vi "UHR-Fleezers Control (host) - 12.5.vi"() -> ()   [LabVIEW 2012] (continued)
            n989 = call "Set Stage Position.vi"("Position"=w1420, "error in"=w1421, "VISA resource name in"=w1422) -> ()  [unwired: 3 out]
          }
          frame #3 {
            # "stop saving"
            n990 = local write "Stop Saving"(TRUE ("Stop Saving")) -> ()
            n991 = local write "Stage Moving"(FALSE ("Stage Moving")) -> ()
          }
        }
      }
      event "Move to Position 1", "Move to Position 2", "Move to Position 3", "Move to Position 4", "Move to Position 5", "Lower Ch. Cap.": Value Change {
        n992 = event-data() -> ()  [unwired: 1 in, 5 out]
        n993 = Or(x="Move to Position 5", y="Lower Ch. Cap.") -> (x .or. y?=w1428:bool)
        n994 = Build Array("Move to Position 1", "Move to Position 2", "Move to Position 3", "Move to Position 4", w1428) -> (w1431:bool[])
        n995 = Boolean Array To Number(Boolean array=w1431) -> (number=w1430:u32)
        n996 = Logarithm Base 2(1:w1430) -> (0:w1429:dbl)
        n997 = flat-sequence {
          tunnel: w1429 -> [w1440]
          tunnel: w1426 -> [w1438]
          tunnel: w1425 -> [w1437]
          frame #0 {
            n998 = local read "Saved Stage Positions"() -> (w1448:dbl[][])
            n999 = Array Subset(array=w1448, index (row)=w1440, length (row)=1 ("length"), index (col)=1 ("index"), length (col)=3 ("length")) -> (w1445:dbl[][])
            n1000 = Reshape Array(w1445, 3 ("dimension size")) -> (w1443:dbl[])
            n1001 = Array To Cluster(array=w1443) -> (cluster=w1442:cluster{"[0]":dbl, "[1]":dbl, "[2]":dbl})
            n1002 = call "Set Stage Position.vi"("Position"=w1442, "error in"=w1437, "VISA resource name in"=w1438) -> ("error out"=w1441:errorcluster)  [unwired: 2 out]
            n1003 = local write "Stage Moving"(TRUE ("Stage Moving")) -> ()
            n1004 = local write "Stage Control Serial Error"(w1441) -> ()
          }
          frame #1 {
            n1005 = local write "Stage Moving"(FALSE ("Stage Moving")) -> ()
            n1006 = call <vilib>:"Beep.vi"() -> ()  [unwired: 3 in, 9 out]
          }
        }
      }
      event "Got ADig bead": Value Change {
        n1007 = event-data() -> ()  [unwired: 1 in, 5 out]
        n1008 = flat-sequence {
          frame #0 {
            n1009 = local read "Cap 1 Samp Flow ON"() -> (w1452:bool)
            n1010 = case shown="True" w1452 {
              frame False {
              }
              frame True {
                n1011 = property on="Sample Channel\nFlow" class="Bool (strict)"("Val(Sgnl)"=TRUE ("Value (Signaling)")) -> ()  [unwired: 2 in, 2 out]
              }
            }
          }
          frame #1 {
            n1012 = property on="Inject Pump 3" class="Bool (strict)"("Val(Sgnl)"=FALSE ("Value (Signaling)")) -> ()  [unwired: 2 in, 2 out]
          }
          frame #2 {
            n1013 = property on="Move Cap. 1 (DNA Bottom)" class="Bool (strict)"("Val(Sgnl)"=TRUE ("Value (Signaling)")) -> ()  [unwired: 2 in, 2 out]
          }
        }
      }
      event "Force FB Data\nScript": Value Change {
        n1014 = event-data() -> ()  [unwired: 1 in, 5 out]
        n1015 = flat-sequence {
          tunnel: w1461 -> [w1465]
          tunnel: w1462 -> [w1466]
          tunnel: [w1466] -> w1457
          tunnel: [w1465] -> w1456
          tunnel: w1457 -> [w1469]
          tunnel: w1456 -> [w1468]
          tunnel: ["Trap Trig Fl."] -> w1458
          tunnel: [w1494] -> w1459
          tunnel: w1458 -> [w1494]
          tunnel: [w1498] -> w1460
          tunnel: w1459 -> [w1498]
          tunnel: w1460 -> [w1500]
          frame #0 {
            n1016 = property on="Trap Delta (MHz)" class="DigNum (strict)"("Val(Sgnl)"="Trap Delta Before Moving") -> ()  [unwired: 2 in, 2 out]
          }
          frame #1 {
            n1017 = local read "Saved Stage Positions"() -> (w1471:dbl[][])
            n1018 = local write "FB Trap Pos Offset"(0.0 ("FB Trap Pos Offset")) -> ()
            n1019 = property on="Trap Pos. FB Offset Factor" class="DigNum (strict)"("Val(Sgnl)"=i64 0 ("Value (Signaling)")) -> ()  [unwired: 2 in, 2 out]
            n1020 = local write "Stage Moving"(TRUE ("Stage Moving")) -> ()
            n1021 = call "move to saved stage position.vi"("error in"=w1468, "Stage VISA resource name in"=w1469, "Position"="Stage Position To Establish FB", "Saved Stage Positions"=w1471) -> ("error out"=w1467:errorcluster)  [unwired: 1 out]
            n1022 = local write "Stage Control Serial Error"(w1467) -> ()
          }
          frame #2 {
            n1023 = call <vilib>:"Beep.vi"() -> ()  [unwired: 3 in, 9 out]
            n1024 = Multiply(x="Wait (s)", y=u32 1000 ("milliseconds to wait")) -> (x*y=w1478:u32)
            n1025 = property on="Trap Delta (MHz)" class="DigNum (strict)"("Val(Sgnl)"="Starting \nTrap Delta (MHz)") -> ()  [unwired: 2 in, 2 out]
            n1026 = local write "Stage Moving"(FALSE ("Stage Moving")) -> ()
            n1027 = Wait (ms)(milliseconds to wait=w1478) -> ()  [unwired: 1 out]
            n1028 = property on="Tab Control 2" class="TabCtl (strict)"("Val(Sgnl)"=T6."Feedback on Trap Position" ("Value (Signaling)")) -> ()  [unwired: 2 in, 2 out]
            n1029 = property on="Tab Control" class="TabCtl (strict)"("Val(Sgnl)"=T4."Trap Control (RF)" ("Value (Signaling)")) -> ()  [unwired: 2 in, 2 out]
          }
          frame #3 {
            n1030 = property on="Set Reading to\nSetpoint" class="Bool (strict)"("Val(Sgnl)"=TRUE ("Value (Signaling)")) -> ()  [unwired: 2 in, 2 out]
            n1031 = Wait (ms)(milliseconds to wait=u32 500) -> ()  [unwired: 1 out]
          }
          frame #4 {
            n1032 = property on="Trap Pos. FB ON" class="Bool (strict)"("Val(Sgnl)"=TRUE ("Value (Signaling)")) -> ()  [unwired: 2 in, 2 out]
            n1033 = Wait (ms)(milliseconds to wait=u32 250) -> ()  [unwired: 1 out]
          }
          frame #5 {
            n1034 = case shown="False" "Trap Trig Fl." {
              frame False {
                n1035 = case shown="True" "Green ON after FB ON?" {
                  selector: "Green ON after FB ON?" -> [_ w1493]
                  frame False {
                  }
                  frame True {
                    n1036 = property on="Green Laser ON" class="Bool (strict)"("Val(Sgnl)"=w1493) -> ()  [unwired: 2 in, 2 out]
                  }
                }
              }
              frame True {
              }
            }
            n1037 = case shown="True" "Remove Action Offset" {
              tunnel: TRUE ("Value (Signaling)") -> [w1490 w1491]
              frame False {
                n1038 = property on="Remove Unwinding Offset" class="Bool (strict)"("Val(Sgnl)"=w1490) -> ()  [unwired: 2 in, 2 out]
              }
              frame True {
                n1039 = property on="Remove Action Offset" class="Bool (strict)"("Val(Sgnl)"=w1491) -> ()  [unwired: 2 in, 2 out]
              }
            }
            n1040 = Wait (ms)(milliseconds to wait=u32 250) -> ()  [unwired: 1 out]
          }
          frame #6 {
            n1041 = property on="Start Saving" class="Bool (strict)"("Val(Sgnl)"=TRUE ("Value (Signaling)")) -> ()  [unwired: 2 in, 2 out]
            n1042 = Wait (ms)(milliseconds to wait=u32 5000) -> ()  [unwired: 1 out]
          }
          frame #7 {
            w1497 = TRUE ("Value (Signaling)")
            n1043 = property on="Rem fb disp offset" class="Bool (strict)"("Val(Sgnl)"=w1497) -> ()  [unwired: 2 in, 2 out]
            n1044 = property on="Remove Offset" class="Bool (strict)"("Val(Sgnl)"=w1497) -> ()  [unwired: 2 in, 2 out]
            n1045 = Wait (ms)(milliseconds to wait=u32 100) -> ()  [unwired: 1 out]
          }
          frame #8 {
            n1046 = case shown="True" w1500 {
              frame False {
              }
              frame True {
                n1047 = local write "Trap Trig. Fl."(TRUE ("Value (Signaling)")) -> ()
              }
            }
          }
          frame #9 {
            n1048 = case shown="True" "Start dipping after?" {
              frame False {
              }
              frame True {
                n1049 = flat-sequence {
                  frame #0 {
                    n1050 = Multiply(x="Delay before dipping (s)", y=1000.0) -> (x*y=w1504:dbl)
                    n1051 = Wait (ms)(milliseconds to wait=w1504) -> ()  [unwired: 1 out]
                  }
                  frame #1 {
                    n1052 = property on="Dip for Protein" class="Bool (strict)"("Val(Sgnl)"=TRUE ("Value (Signaling)")) -> ()  [unwired: 2 in, 2 out]
                    n1053 = local write "Scripts"(T1."Dipping" ("Scripts")) -> ()
                  }
                }
              }
            }
          }
        }
      }
      event "Fixed Traps Data\nScript": Value Change {
        n1054 = event-data() -> ()  [unwired: 1 in, 5 out]
        n1055 = flat-sequence {
          frame #0 {
            n1056 = case shown="True" "Green ON" {
              frame False {
              }
              frame True {
                n1057 = property on="Green Laser ON" class="Bool (strict)"("Val(Sgnl)"=TRUE) -> ()  [unwired: 2 in, 2 out]
              }
            }
            n1058 = local write "Offset (nm)"(0.0 ("Offset (nm)")) -> ()
            n1059 = property on="Sample Channel\nFlow" class="Bool (strict)"("Val(Sgnl)"=FALSE ("Value (Signaling)")) -> ()  [unwired: 2 in, 2 out]
            n1060 = property on="Trap Delta (MHz)" class="DigNum (strict)"("Val(Sgnl)"="Fixed Traps Trap Delta (MHz)") -> ()  [unwired: 2 in, 2 out]
          }
          frame #1 {
            n1061 = Wait (ms)(milliseconds to wait=u32 1000) -> ()  [unwired: 1 out]
          }
          frame #2 {
            n1062 = local write "Start Saving"(TRUE ("Start Saving")) -> ()
          }
          frame #3 {
            n1063 = local read "Bead Sep. Int. Time (s)"() -> (w1515:dbl)
            n1064 = Multiply(x=w1515, y=1000.0) -> (x*y=w1517:dbl)
            n1065 = Wait (ms)(milliseconds to wait=w1517) -> ()  [unwired: 1 out]
          }
          frame #4 {
            n1066 = property on="Remove Offset" class="Bool (strict)"("Val(Sgnl)"=TRUE ("Value (Signaling)")) -> ()  [unwired: 2 in, 2 out]
          }
          frame #5 {
            n1067 = property on="Dip for Protein" class="Bool (strict)"("Val(Sgnl)"="Start dipping after?") -> ()  [unwired: 2 in, 2 out]
          }
        }
      }
      event "Got DNA bead": Value Change {
        n1068 = event-data() -> ()  [unwired: 1 in, 5 out]
        n1069 = flat-sequence {
          frame #0 {
            n1070 = local read "Daq spot flow on"() -> (w1522:bool)
            n1071 = case shown="True" w1522 {
              frame False {
              }
              frame True {
                n1072 = property on="Sample Channel\nFlow" class="Bool (strict)"("Val(Sgnl)"=TRUE ("Value (Signaling)")) -> ()  [unwired: 2 in, 2 out]
              }
            }
            n1073 = property on="Got DNA bead" class="Bool"("Key Focus"=FALSE) -> ()  [unwired: 2 in, 2 out]
          }
          frame #1 {
            n1074 = property on="Inject Pump 1" class="Bool (strict)"("Val(Sgnl)"=FALSE ("Value (Signaling)")) -> ()  [unwired: 2 in, 2 out]
          }
          frame #2 {
            n1075 = property on="Cal/Data Acq. Spot" class="Bool (strict)"("Val(Sgnl)"=TRUE ("Value (Signaling)")) -> ()  [unwired: 2 in, 2 out]
          }
        }
      }
      event "Take Stepping Data": Value Change {
        n1076 = event-data() -> ()  [unwired: 1 in, 5 out]
        n1077 = local read "Save ave N"() -> (w1534:dbl)
        n1078 = flat-sequence {
          tunnel: w1534 -> [w1536]
          tunnel: [w1536] -> w1529
          tunnel: [w1538] -> w1530
          tunnel: w1529 -> [w1538]
          tunnel: [w1540] -> w1531
          tunnel: w1530 -> [w1540]
          tunnel: [w1543] -> w1532
          tunnel: w1531 -> [w1543]
          tunnel: [w1545] -> w1533
          tunnel: w1532 -> [w1545]
          tunnel: [w1547] -> w1527
          tunnel: w1533 -> [w1547]
          tunnel: w1527 -> [w1550]
          tunnel: [w1550] -> w1526
          tunnel: w1526 -> [w1551]
          tunnel: [w1551] -> w1528
          tunnel: w1528 -> [w1557]
          frame #0 {
            n1079 = property on="Save ave N" class="DigNum (strict)"("Val(Sgnl)"="Save ave factor") -> ()  [unwired: 2 in, 2 out]
          }
          frame #1 {
            n1080 = Wait (ms)(milliseconds to wait=u32 100) -> ()  [unwired: 1 out]
          }
          frame #2 {
            n1081 = local read "Offset 2 Start (MHz)"() -> (w1542:dbl)
            n1082 = property on="Saved AOD Raster Scan Parameter Sets" class="Arr (strict)"("Index Values"=u32[] [2]) -> ()  [unwired: 2 in, 2 out]
            n1083 = property on="Trap Delta (MHz)" class="DigNum (strict)"("Val(Sgnl)"=w1542) -> ()  [unwired: 2 in, 2 out]
          }
          frame #3 {
            n1084 = property on="Load parameters" class="Bool (strict)"("Val(Sgnl)"=TRUE ("Value (Signaling)")) -> ()  [unwired: 2 in, 2 out]
          }
          frame #4 {
            n1085 = Wait (ms)(milliseconds to wait=u32 100) -> ()  [unwired: 1 out]
          }
          frame #5 {
            n1086 = property on="Trap Raster Scan" class="Bool (strict)"("Val(Sgnl)"=TRUE ("Value (Signaling)")) -> ()  [unwired: 2 in, 2 out]
          }
          frame #6 {
            n1087 = Wait (ms)(milliseconds to wait=u32 1000) -> ()  [unwired: 1 out]
          }
          frame #7 {
            n1088 = while {
              stop <- w1554 stop-if-true
              n1089 = local read "Raster Scanning..."() -> (w1556:bool)
              n1090 = local read "Saving..."() -> (w1555:bool)
              n1091 = Not(x=w1555) -> (.not. x?=w1552:bool)
              n1092 = Not(x=w1556) -> (.not. x?=w1553:bool)
              n1093 = And(x=w1553, y=w1552) -> (x .and. y?=w1554:bool)
            }
          }
          frame #8 {
            n1094 = property on="Save ave N" class="DigNum (strict)"("Val(Sgnl)"=w1557) -> ()  [unwired: 2 in, 2 out]
          }
        }
      }
      event "Step Size (nm)": Value Change {
        n1095 = event-data() -> ()  [unwired: 1 in, 5 out]
        n1096 = flat-sequence {
          frame #0 {
            n1097 = property on="Saved AOD Raster Scan Parameter Sets" class="Arr (strict)"("Index Values"=u32[] [1]) -> ()  [unwired: 2 in, 2 out]
          }
          frame #1 {
            n1098 = Multiply(x="N Steps", y="Step Size (nm)") -> (x*y=w1559:dbl)
            n1099 = property on="Scan Speed AOD (nm/s) 2" class="DigNum (strict)"("Value"="Step Size (nm)") -> ()  [unwired: 2 in, 2 out]
            n1100 = property on="Step Size AOD (nm) 2" class="DigNum (strict)"("Value"="Step Size (nm)") -> ()  [unwired: 2 in, 2 out]
            n1101 = property on="Scan Range AOD (nm) 2" class="DigNum (strict)"("Value"=w1559) -> ()  [unwired: 2 in, 2 out]
          }
        }
      }
      event "Take Detection Laser\nImage": Value Change {
        n1102 = event-data() -> ()  [unwired: 1 in, 5 out]
        n1103 = flat-sequence {
          tunnel: [w1587] -> w1577
          tunnel: [w1586] -> w1570
          tunnel: [w1585] -> w1562
          tunnel: [w1590] -> w1578
          tunnel: w1577 -> [w1590]
          tunnel: [w1589] -> w1571
          tunnel: w1570 -> [w1589]
          tunnel: [w1588] -> w1563
          tunnel: w1562 -> [w1588]
          tunnel: [w1594] -> w1579
          tunnel: w1578 -> [w1594]
          tunnel: [w1593] -> w1572
          tunnel: w1571 -> [w1593]
          tunnel: [w1592] -> w1564
          tunnel: w1563 -> [w1592]
          tunnel: [w1600] -> w1580
          tunnel: w1579 -> [w1600]
          tunnel: [w1599] -> w1573
          tunnel: w1572 -> [w1599]
          tunnel: [w1598] -> w1565
          tunnel: w1564 -> [w1598]
          tunnel: [w1604] -> w1581
          tunnel: w1580 -> [w1604]
          tunnel: [w1603] -> w1574
          tunnel: w1573 -> [w1603]
          tunnel: [w1602] -> w1566
          tunnel: w1565 -> [w1602]
          tunnel: [w1608] -> w1582
          tunnel: w1581 -> [w1608]
          tunnel: [w1607] -> w1575
          tunnel: w1574 -> [w1607]
          tunnel: [w1606] -> w1567
          tunnel: w1566 -> [w1606]
          tunnel: [w1612] -> w1583
          tunnel: w1582 -> [w1612]
          tunnel: [w1611] -> w1576
          tunnel: w1575 -> [w1611]
          tunnel: [w1610] -> w1568
          tunnel: w1567 -> [w1610]
          tunnel: w1583 -> [w1618]
          tunnel: w1576 -> [w1617]
          tunnel: [w1615] -> w1569
          tunnel: w1568 -> [w1615]
          tunnel: w1569 -> [w1619]
          frame #0 {
            n1104 = local read "Laser interlacing mode"() -> (w1586:enum32{"Laser ON", "Laser OFF", "Interlace"})
            n1105 = local read "Green FB On/Off"() -> (w1585:bool)
            n1106 = local read "Green Laser ON"() -> (w1587:bool)
          }
          frame #1 {
            n1107 = property on="Green FB On/Off" class="Bool (strict)"("Val(Sgnl)"=FALSE ("Value (Signaling)")) -> ()  [unwired: 2 in, 2 out]
          }
          frame #2 {
            n1108 = property on="Green Laser ON" class="Bool (strict)"("Val(Sgnl)"=TRUE ("Value (Signaling)")) -> ()  [unwired: 2 in, 2 out]
            n1109 = property on="Flip Green Filter" class="Bool (strict)"("Val(Sgnl)"=TRUE ("Value (Signaling)")) -> ()  [unwired: 2 in, 2 out]
            n1110 = property on="Laser interlacing mode" class="RadioBtnsControl (strict)"("Val(Sgnl)"=enum32{"Laser ON", "Laser OFF", "Interlace"}."Laser ON" ("Value (Signaling)")) -> ()  [unwired: 2 in, 2 out]
          }
          frame #3 {
            n1111 = Wait (ms)(milliseconds to wait=u32 500) -> ()  [unwired: 1 out]
          }
          frame #4 {
            n1112 = property on="Confocal Image" class="Bool (strict)"("Val(Sgnl)"=TRUE ("Value (Signaling)")) -> ()  [unwired: 2 in, 2 out]
          }
          frame #5 {
            n1113 = Wait (ms)(milliseconds to wait=u32 2000) -> ()  [unwired: 1 out]
          }
          frame #6 {
            n1114 = while {
              stop <- w1613 stop-if-true
              n1115 = local read "Saving..."() -> (w1614:bool)
              n1116 = Not(x=w1614) -> (.not. x?=w1613:bool)
            }
          }
          frame #7 {
            n1117 = property on="Flip Green Filter" class="Bool (strict)"("Val(Sgnl)"=TRUE ("Value (Signaling)")) -> ()  [unwired: 2 in, 2 out]
            n1118 = property on="Green Laser ON" class="Bool (strict)"("Val(Sgnl)"=w1618) -> ()  [unwired: 2 in, 2 out]
            n1119 = property on="Laser interlacing mode" class="RadioBtnsControl (strict)"("Val(Sgnl)"=w1617) -> ()  [unwired: 2 in, 2 out]
          }
          frame #8 {
            n1120 = property on="Green FB On/Off" class="Bool (strict)"("Val(Sgnl)"=w1619) -> ()  [unwired: 2 in, 2 out]
          }
        }
      }
      event "Stop All": Value Change {
        n1121 = event-data() -> ()  [unwired: 1 in, 5 out]
        n1122 = local read "Delay (ms)"() -> (w1622:i32)
        n1123 = call "serial write macro.vi"("String"="l0", "Delay (ms)"=w1622, "VISA resource name"=w1625) -> ("read buffer"=w1620:string, "error out"=w1621:errorcluster, "VISA resource name out"=w1624:refnum<visa-resource-name>)
        n1124 = local write "read blue buffer"(w1620) -> ()
        n1125 = local write "Blue Error Out"(w1621) -> ()
        n1126 = VISA Close(VISA resource name=w1624) -> ()  [unwired: 1 in, 1 out]
        n1127 = local read "Stop All"() -> (w1626:bool)
      }
    }
    n1128 = node-c288() -> ()  [unwired: 1 in, 1 out]
  }
  n1129 = timed-loop "Basic control parameters (all FPGA settings, other basic controls)" {
    tunnel: w13 -> [w1635]
    shift-right: [w1634] -> _
    shift-left: errorcluster {"status"=FALSE, "code"=0, "source"=""} ("error out") -> [w1633]
    tunnel: [w1632] -> _
    timing: w127 -> [_]
    timing-out: [_] -> w126
    tunnel: w100 -> [w1631]
    tunnel: w72 -> [w1630]
    tunnel: w71 -> [w1629]
    tunnel: w70 -> [w1628]
    tunnel: w69 -> [w1627]
    stop <- w1632 stop-if-true
    n1130 = node-c288() -> ()  [unwired: 2 out]
    n1131 = event shown="[0] \"AI Count (ticks)\", \"Sets to FIFO (Traps)\", \"Save ave N\", \"FPGA Ave.\", \"# Samples/channel\", \"N sets to save\": Value Change" {
      selector: _ -> [_ _ _ _ _ _ _ _ _ _ _ _ _ _ _ _ _ _ _ _ _ _ _ _ _ _ _ _ _ _ _ _ _ _ _ _ _ _ _ _ _ _ _ _ _ _ _ _ _ _ _ _ _ _ _ _ _ _ _ _ _ _ _ _ _ _ _ _ _ _ _ _ _ _]
      dyn-events: _ -> [_ _ _ _ _ _ _ _ _ _ _ _ _ _ _ _ _ _ _ _ _ _ _ _ _ _ _ _ _ _ _ _ _ _ _ _ _ _ _ _ _ _ _ _ _ _ _ _ _ _ _ _ _ _ _ _ _ _ _ _ _ _ _ _ _ _ _ _ _ _ _ _ _ _]
      timeout: _ -> [_ _ _ _ _ _ _ _ _ _ _ _ _ _ _ _ _ _ _ _ _ _ _ _ _ _ _ _ _ _ _ _ _ _ _ _ _ _ _ _ _ _ _ _ _ _ _ _ _ _ _ _ _ _ _ _ _ _ _ _ _ _ _ _ _ _ _ _ _ _ _ _ _ _]
      tunnel: w1635 -> [w1676 _ _ _ w1714 _ w1736 _ _ _ _ w1802 _ _ w1845 w1851 w1858 w1863 w1954 _ w1970 w1995 w2016 w2037 w2058 w2087 w2113 w2116 w2120 w2215 w2220 w2258 _ w2293 w2297 w2308 w2312 w2316 _ w2324 _ _ _ _ _ _ _ _ _ _ _ _ _ _ _ _ _ w2702 _ w2719 _ w2726 w2744 _ w2751 w2759 w2774 w2790 w2796 _ w2805 _ w2824 _]
      tunnel: [w1675 _ _ _ w1704 _ w1735 _ _ w1767 _ w1781 _ _ w1844 w1847 w1857 w1860 w1948 _ w1969 w1994 w2014 w2035 w2056 w2081 w2111 _ w2118 w2213 w2218 w2256 _ w2291 w2295 w2299 w2310 w2314 _ w2322 _ _ _ _ _ _ _ _ _ _ _ _ _ _ _ _ _ w2700 _ _ _ _ w2741 _ _ _ _ _ _ _ _ _ _ _] -> w1634
      tunnel: w1633 -> [w1674 _ _ _ w1713 _ w1734 _ _ w1767 _ w1801 _ _ w1843 w1846 w1856 w1859 w1953 _ w1968 w1993 w2015 w2036 w2057 w2086 w2112 w2115 w2119 w2214 w2219 w2257 _ w2292 w2296 w2307 w2311 w2315 _ w2323 _ _ _ _ _ _ _ _ _ _ _ _ _ _ _ _ _ w2701 _ w2718 _ w2725 w2743 _ w2750 w2758 w2773 w2789 w2795 _ w2804 _ w2823 _]
      tunnel: [_ _ _ _ _ _ _ _ _ w1766 _ _ _ _ _ _ _ _ _ _ _ _ _ _ _ _ _ _ _ _ _ _ _ _ _ _ _ _ _ _ _ _ _ _ _ _ _ _ _ _ _ _ _ _ _ _ _ _ _ _ _ _ _ _ _ _ _ _ _ _ _ _ _ _] -> w1632
      tunnel: [_ _ _ _ _ _ _ "Round T1 X" _ _ _ _ _ _ _ _ _ _ _ _ _ _ _ _ _ _ _ _ _ _ _ _ _ _ _ _ _ _ _ _ _ _ _ _ _ _ _ _ _ _ _ _ _ _ _ _ _ _ _ _ _ _ _ _ _ _ _ _ _ _ _ _ _ _] -> _
      tunnel: [_ _ _ "Adjust Scale\nto Mean" _ _ _ _ _ _ _ _ _ _ _ _ _ _ _ _ _ _ _ _ _ _ _ _ "Test ttrig" _ _ _ _ _ _ _ _ _ _ _ _ _ _ _ _ _ _ "Flush Sample" "Flush Pump 3" "Flush Pump 1" "Clear Volume" _ _ _ _ _ _ _ _ _ _ _ _ _ _ _ _ _ _ _ _ _ _ _] -> _
      tunnel: [_ _ _ _ _ _ _ _ "Round T2 X" _ "Delayed Interlace Start" _ _ _ _ _ _ _ _ _ _ _ _ _ _ _ _ _ _ _ _ _ _ _ _ _ _ _ _ _ _ _ _ _ _ _ _ _ _ _ _ _ _ _ _ _ _ _ _ _ _ _ _ _ _ _ _ _ _ _ _ _ _ _] -> _
      tunnel: w1631 -> [_ _ _ _ _ _ _ _ _ _ _ _ _ _ _ _ _ _ _ _ _ _ _ _ _ _ _ _ _ _ _ _ _ _ _ _ _ _ _ _ _ _ _ w2481 w2488 w2495 w2500 w2509 _ _ w2615 _ _ _ _ _ _ _ _ _ _ _ _ _ _ _ _ _ _ _ _ _ _ _]
      tunnel: w1630 -> [_ _ _ _ _ _ _ _ _ _ _ _ _ _ _ _ _ _ _ _ _ _ _ _ _ _ _ _ _ _ _ _ _ _ _ _ _ _ _ _ _ w2398 _ _ _ _ _ _ w2553 _ _ w2621 _ w2630 _ w2644 _ _ _ _ _ _ _ _ _ _ _ _ _ _ _ _ _ _]
      tunnel: w1629 -> [_ _ _ _ _ _ _ _ _ _ _ _ _ _ _ _ _ _ _ _ _ _ _ _ _ _ _ _ _ _ _ _ _ _ _ _ _ _ _ _ _ _ _ _ _ _ _ _ _ _ _ _ _ _ _ _ _ _ _ _ _ _ _ _ _ _ _ _ _ _ _ _ _ _]
      tunnel: w1628 -> [_ _ _ _ _ _ _ _ _ _ _ _ _ _ _ _ _ _ _ _ _ _ _ _ _ _ _ _ _ _ _ _ _ _ _ _ _ _ _ _ w2335 _ _ _ _ _ _ _ _ w2583 _ _ w2626 _ w2637 _ w2669 _ _ _ _ _ _ _ _ _ _ _ _ _ _ _ _ _]
      tunnel: w1627 -> [_ _ _ _ _ _ _ _ _ _ _ _ _ _ _ _ _ _ _ _ _ _ _ _ _ _ _ _ _ _ _ _ _ _ _ _ _ _ _ _ _ _ _ _ _ _ _ _ _ _ _ _ _ _ _ _ _ _ _ _ _ _ _ _ _ _ _ _ _ _ _ _ _ _]
      event "AI Count (ticks)", "Sets to FIFO (Traps)", "Save ave N", "FPGA Ave.", "# Samples/channel", "N sets to save": Value Change {
        # "So that if 'Save ave N' is updated, the AOD scanning code updates too."
        n1132 = event-data() -> ()  [unwired: 6 out]
        n1133 = local read "AI Count (ticks)"() -> (w1658:u16)
        n1134 = Unbundle By Name("Sets to FIFO (Traps)") -> ("Set 1"=w1641:bool, "Set 2"=w1640:bool, "Set 3"=w1639:bool)
        n1135 = Boolean To (0,1)(Boolean="Sets to FIFO (Traps)") -> (0, 1=w1666:cluster{"Set 1":i16, "Set 2":i16, "Set 3":i16})
        n1136 = xnode "Read/Write Control"("FPGA VI Reference In"=w1676, "error in"=w1674, "ai count"=w1658, "Set 1"=w1641, "Set 2"=w1640, "Set 3"=w1639, "N of AI1 Int Acq Sets"="N Acq Sets (Traps + Fl.)") -> ("error out"=w1675:errorcluster)  [unwired: 1 out]
        n1137 = Cluster To Array(cluster=w1666) -> (array=w1665:i16[])
        n1138 = To Unsigned Long Integer(number=w1665) -> (unsigned 32bit integer=w1647:u32[])
        n1139 = local read "Scan steps (AOD)"() -> (w1667:u64)
        n1140 = Multiply(x=w1658, y="N Acq Sets (Traps + Fl.)") -> (x*y=w1656:u16)
        n1141 = Divide(x=40000000.0, y=w1658) -> (x/y=w1650:dbl)
        "AI rate (Hz)" <- w1650
        "Ave. Rate (Hz)" <- w1650
        n1142 = Add Array Elements(numeric array=w1647) -> (sum=w1659:u32)
        "Trap Sets" <- w1659
        n1143 = Reciprocal(x=w1650) -> (1/x=→"Ave. Period (s)":dbl)
        n1144 = property on="Scan steps (AOD)" class="DigNum (strict)"("Val(Sgnl)"=w1667) -> ()  [unwired: 2 in, 2 out]
        n1145 = Divide(x=w1650, y="N Acq Sets (Traps + Fl.)") -> (x/y=w1671:dbl)
        "Data Rate (Hz)" <- w1671
        n1146 = Reciprocal(x=w1671) -> (1/x=→"Data Period (s)":dbl)
        n1147 = local read "Save ave N"() -> (w1670:dbl)
        n1148 = Divide(x=w1671, y=w1670) -> (x/y=w1669:dbl)
        "Save Data Rate (Hz)" <- w1669
        n1149 = Reciprocal(x=w1669) -> (1/x=→"Save Data Period (s)":dbl)
        n1150 = Multiply(x=w1656, y="# Samples/trap") -> (x*y=w1654:u32)
        "Counts/DMA" <- w1654
        n1151 = property on="Trap Disp. Downsample" class="DigNum (strict)"("Maximum"="# Samples/trap") -> ()  [unwired: 2 in, 2 out]
        n1152 = Multiply(x=w1659, y="# Samples/trap") -> (x*y=w1648:u32)
        "# Samples/channel" <- w1648
        n1153 = Multiply(x=w1648, y=u32 8) -> (x*y=→"Trap AI Elements/DMA read":u32)
        n1154 = local read "APD Int. Count"() -> (w1655:u32)
        n1155 = Multiply(x=w1648, y=u32 3) -> (x*y=→"Trap Pos Elements/DMA read":u32)
        n1156 = Divide(x=w1654, y=w1655) -> (x/y=w1645:dbl)
        "APD Samples/FIFO Acq." <- w1645
        n1157 = Divide(x=w1654, y=40000000.0) -> (x/y=w1652:dbl)
        "DMA Update Period (s)" <- w1652
        n1158 = local read "Number of APDs"() -> (w1638:u8)
        n1159 = Multiply(x=w1638, y=w1645) -> (x*y=→"APD Elements/DMA read":dbl)
        n1160 = property on="APD Disp. Downsample" class="DigNum (strict)"("Maximum"=w1645) -> ()  [unwired: 2 in, 2 out]
        n1161 = local read "N sets to save"() -> (w1664:u32)
        n1162 = Multiply(x=w1652, y=w1664) -> (x*y=→"Total Time (s)":dbl)
        "FPGA Averaging" <- FALSE ("FPGA Averaging")
      }
      event "Remove Offset": Value Change {
        n1163 = event-data() -> ()  [unwired: 7 out]
        n1164 = local write "Remove Offset"(FALSE ("Remove Offset")) -> ()
        n1165 = local read "Bead Mean (nm)"() -> (w1678:dbl)
        n1166 = local read "Offset (nm)"() -> (w1679:dbl)
        n1167 = Add(x=w1678, y=w1679) -> (x+y=w1677:dbl)
        n1168 = local write "Offset (nm)"(w1677) -> ()
        n1169 = disable-structure shown="Disabled" {
          frame Disabled {
            n1170 = local read "Bead Mean (nm)"() -> (w1684:dbl)
            n1171 = Add(y=w1684) -> (x=w1683:dbl, x+y=w1682:dbl)
            n1172 = Subtract(x=w1684, y=w1683) -> (x-y=w1681:dbl)
            n1173 = property on="Bead Separation" class="WFChart (strict)"("YScale.Minimum"=w1681) -> ()  [unwired: 2 in, 2 out]
            n1174 = property on="Bead Separation" class="WFChart (strict)"("YScale.Maximum"=w1682) -> ()  [unwired: 2 in, 2 out]
          }
          frame Enabled {
          }
        }
      }
      event "Detector Type": Value Change {
        n1175 = event-data() -> ()  [unwired: 7 out]
        n1176 = local read "AI labels"() -> (w1685:string[])
        n1177 = property on="High Res. Display" class="Ring (strict)"("Strings []"=w1685) -> ()  [unwired: 2 in, 2 out]
        n1178 = Build Array (concatenate)(w1685, "none") -> (w1686:string[])
        n1179 = property on="FFT 1 Choice 1" class="Ring (strict)"("Strings []"=w1686) -> ()  [unwired: 2 in, 2 out]
        n1180 = property on="FFT 1 Choice 2" class="Ring (strict)"("Strings []"=w1686) -> ()  [unwired: 2 in, 2 out]
        n1181 = property on="FFT 2 Choice 1" class="Ring (strict)"("Strings []"=w1686) -> ()  [unwired: 2 in, 2 out]
        n1182 = property on="FFT 2 Choice 2" class="Ring (strict)"("Strings []"=w1686) -> ()  [unwired: 2 in, 2 out]
        n1183 = Bundle("APD 1", "APD 2") -> (w1689:cluster{string, string})  [unwired: 1 out]
        n1184 = Cluster To Array(cluster=w1689) -> (array=w1687:string[])
        n1185 = Build Array (concatenate)(w1687, w1686) -> (w1691:string[])
        n1186 = Array Size(array=w1691) -> (size(s)=w1692:i32)
        n1187 = property on="Signals to Plot" class="LstBox (strict)"("Item Names"=w1691) -> ()  [unwired: 2 in, 2 out]
        n1188 = property on="Signals to Plot" class="LstBox (strict)"("Number of Rows"=w1692) -> ()  [unwired: 2 in, 2 out]
        n1189 = property on="All Signals" class="WFChart (strict)"("LegNumRows"=w1692) -> ()  [unwired: 2 in, 2 out]
      }
      event "Adjust Scale\nto Mean": Value Change {
        n1190 = event-data() -> ()  [unwired: 7 out]
        n1191 = local read "APD 1 Rate (Hz)"() -> (w1701:dbl)
        n1192 = Multiply(x=1000.0, y="Above (kHz)") -> (x*y=w1699:dbl)
        n1193 = Multiply(x=1000.0, y="Below (kHz)") -> (x*y=w1697:dbl)
        n1194 = Add(x=w1699, y=w1701) -> (x+y=w1694:dbl)
        n1195 = Subtract(x=w1701, y=w1697) -> (x-y=w1695:dbl)
        n1196 = property on="APD Chart" class="WFChart (strict)"("YScale.Minimum"=w1695) -> ()  [unwired: 2 in, 2 out]
        n1197 = property on="APD Chart" class="WFChart (strict)"("YScale.Maximum"=w1694) -> ()  [unwired: 2 in, 2 out]
      }
      event "Phase adj. (AI1)", "+ phase (AI1)", "- phase (AI1)": Value Change {
        n1198 = event-data() -> ()  [unwired: 7 out]
        n1199 = Negate(x="Phase adj. (AI1)") -> (-x=w1711:i16)
        n1200 = Select(t=w1711, s="- phase (AI1)", f="Phase adj. (AI1)") -> (s? t:f=w1710:i16)
        n1201 = xnode "Read/Write Control"("FPGA VI Reference In"=w1714, "error in"=w1713, "Phase count adjustment"=w1710) -> ("FPGA VI Reference Out"=w1709:T20, "error out"=w1708:errorcluster)
        n1202 = Or(x="- phase (AI1)", y="+ phase (AI1)") -> (x .or. y?=w1705:bool)
        n1203 = xnode "Read/Write Control"("FPGA VI Reference In"=w1709, "error in"=w1708, "+ phase"=w1705) -> ("error out"=w1704:errorcluster)  [unwired: 1 out]
      }
      event "Signals to Plot": Double Click {
        w1717 = u32 9868950 ("Color Box")
        n1204 = event-data() -> ("Row"=w1719:i32)  [unwired: 9 out]
        n1205 = property on="All Signals" class="WFChart (strict)"("Active Plot"=w1719) -> (error out=w1730:errorcluster)  [unwired: 2 in, 1 out]
        n1206 = property on="All Signals" class="WFChart (strict)" props=["Plot", "Visible?", "Plot", "Plot Color"](error in=w1730) -> (error out=w1729:errorcluster, "Plot.Visible?"=w1728:bool)  [unwired: 1 in, 2 out]
        n1207 = Select(t=FALSE ("Plot.Visible"), s=w1728, f=TRUE ("Plot.Visible")) -> (s? t:f=w1723:bool)
        n1208 = property on="All Signals" class="WFChart (strict)"(error in=w1729, "Plot.Visible?"=w1723) -> (error out=w1725:errorcluster)  [unwired: 1 in, 1 out]
        n1209 = property on="All Signals" class="WFChart (strict)"(error in=w1725) -> (error out=w1720:errorcluster, "Plot.Plot Color"=w1724:u32)  [unwired: 1 in, 1 out]
        n1210 = property on="Signals to Plot" class="LstBox (strict)"(error in=w1720, "Active Row"=w1719) -> (error out=w1718:errorcluster)  [unwired: 1 in, 1 out]
        n1211 = Select(t=w1724, s=w1723, f=u32 0) -> (s? t:f=w1721:u32)
        n1212 = property on="Signals to Plot" class="LstBox (strict)"(error in=w1718, "CellFontColor"=w1721, "SelColor"=w1717, "CellBG"=w1717, "CellFontSize"=u32 20 ("Active Row:Cell Font:Size"), "CellFontBold"=TRUE ("Active Row:Cell Font:Bold")) -> ()  [unwired: 1 in, 2 out]
      }
      event "BD 1 Frequency 1 (MHz)", "BD 1 Frequency 2 (MHz)", "BD 1 Frequency 3 (MHz)", "BD 2 Frequency 1 (MHz)", "BD 2 Frequency 2 (MHz)", "BD 2 Frequency 3 (MHz)", "Trap Delta (MHz)": Value Change {
        n1213 = event-data() -> ("CtlRef"=w1733:refnum<vi>)  [unwired: 6 out]
        n1214 = control-ref of="Trap Delta (MHz)"() -> (w1732:refnum<vi>)
        n1215 = Equal?(x=w1732, y=w1733) -> (x = y?=w1731:bool)
        n1216 = case shown="False" "Oscillate Set 1" {
          tunnel: w1736 -> [w1756 _]
          tunnel: [w1755 w1759] -> w1735
          tunnel: w1734 -> [w1754 w1759]
          tunnel: w1731 -> [w1739 _]
          frame False {
            n1217 = local read "BD 1 Frequency 2 (MHz)"() -> (w1743:dbl)
            n1218 = local read "BD 1 Frequency 1 (MHz)"() -> (w1741:dbl)
            n1219 = Subtract(x=w1743, y="Trap Delta (MHz)") -> (x-y=w1740:dbl)
            n1220 = Select(t=w1740, s=w1739, f=w1741) -> (s? t:f=w1738:dbl)
            n1221 = local read "Y RF Frequency Limits (MHz)"() -> (w1744:T16)
            n1222 = local read "X RF Frequency Limits (MHz)"() -> (w1745:T16)
            n1223 = local read "BD 1 Frequency 3 (MHz)"() -> (w1757:dbl)
            n1224 = local write "BD 1 Frequency 1 (MHz)"(w1738) -> ()
            n1225 = local read "BD 2 Frequency 1 (MHz)"() -> (w1748:dbl)
            n1226 = local read "BD 2 Frequency 2 (MHz)"() -> (w1747:dbl)
            n1227 = local read "BD 2 Frequency 3 (MHz)"() -> (w1758:dbl)
            n1228 = call "set RF board frequency - interlace.vi"("Board 2 Frequency Limits"=w1744, "Board 1 Frequency Limits"=w1745, "error in"=w1754, "FPGA VI Reference In"=w1756, "Board 2 Frequency 3 (MHz)"=w1758, "Board 1 Frequency 3 (MHz)"=w1757, "Board 2 Frequency 2 (MHz)"=w1747, "Board 2 Frequency 1 (MHz)"=w1748, "Board 1 Frequency 2 (MHz)"=w1743, "Board 1 Frequency 1  (MHz)"=w1738) -> ("error out"=w1755:errorcluster)  [unwired: 1 out]
            n1229 = Subtract(x=w1748, y=w1747) -> (x-y=w1752:dbl)
            n1230 = Subtract(x=w1738, y=w1743) -> (x-y=w1753:dbl)
            n1231 = Square(x=w1752) -> (x^2=w1750:dbl)
            n1232 = Square(x=w1753) -> (x^2=w1751:dbl)
            n1233 = Add(x=w1751, y=w1750) -> (x+y=w1749:dbl)
            n1234 = Square Root(x=w1749) -> (sqrt(x)=w1746:dbl)
            n1235 = local write "Trap Delta (MHz)"(w1746) -> ()
            n1236 = property on="Initial delta (MHz)" class="DigNum (strict)"("Val(Sgnl)"=w1746) -> ()  [unwired: 2 in, 2 out]
          }
          frame True {
          }
        }
      }
      event "Round T1 X": Value Change {
        n1237 = event-data() -> ()  [unwired: 7 out]
        n1238 = local read "BD 1 Frequency 1 (MHz)"() -> (w1762:dbl)
        n1239 = Round To Nearest(number=w1762) -> (nearest integer value=w1761:dbl)
        n1240 = property on="BD 1 Frequency 1 (MHz)" class="DigNum (strict)"("Val(Sgnl)"=w1761) -> ()  [unwired: 2 in, 2 out]
      }
      event "Round T2 X": Value Change {
        n1241 = event-data() -> ()  [unwired: 7 out]
        n1242 = local read "BD 1 Frequency 2 (MHz)"() -> (w1764:dbl)
        n1243 = Round To Nearest(number=w1764) -> (nearest integer value=w1763:dbl)
        n1244 = property on="BD 1 Frequency 2 (MHz)" class="DigNum (strict)"("Val(Sgnl)"=w1763) -> ()  [unwired: 2 in, 2 out]
      }
      event "Stop All": Value Change {
        n1245 = event-data() -> ()  [unwired: 7 out]
        n1246 = local read "Stop All"() -> (w1766:bool)
      }
      event "Delayed Interlace Start": Value Change {
        n1247 = event-data() -> ()  [unwired: 7 out]
        n1248 = flat-sequence {
          frame #0 {
            n1249 = Multiply(x="Delay to Interlace (s)", y=1000.0) -> (x*y=w1769:dbl)
            n1250 = Wait (ms)(milliseconds to wait=w1769) -> ()  [unwired: 1 out]
          }
          frame #1 {
            n1251 = property on="Laser interlacing mode" class="RadioBtnsControl (strict)"("Val(Sgnl)"=enum32{"Laser ON", "Laser OFF", "Interlace"}."Interlace" ("Value (Signaling)")) -> ()  [unwired: 2 in, 2 out]
          }
        }
      }
      event "BD 1 Amplitude 1 (%)", "BD 1 Amplitude 2 (%)", "BD 1 Amplitude 3 (%)", "BD 2 Amplitude 1 (%)", "BD 2 Amplitude 2 (%)", "BD 2 Amplitude 3 (%)", "Trap 1 ON", "Trap 2 ON", "Trap 3 ON", "Feedback On/Off", "All FB On/Off": Value Change {
        w1793 = i16 1 ("f")
        n1252 = event-data() -> ()  [unwired: 7 out]
        n1253 = local write "Trap 1 (ON/OFF)"("Trap 1 ON") -> ()
        n1254 = local write "Trap 2 (ON/OFF)"("Trap 2 ON") -> ()
        n1255 = Boolean To (0,1)(Boolean="Trap 3 ON") -> (0, 1=w1794:i16)
        n1256 = Boolean To (0,1)(Boolean="Trap 1 ON") -> (0, 1=w1795:i16)
        n1257 = Boolean To (0,1)(Boolean="Trap 2 ON") -> (0, 1=w1796:i16)
        n1258 = Select(t=w1796, s="Trap ON/OFF X or Y Amp?", f=w1793) -> (s? t:f=w1791:i16)
        n1259 = Select(t=w1795, s="Trap ON/OFF X or Y Amp?", f=w1793) -> (s? t:f=w1792:i16)
        n1260 = Select(t=w1794, s="Trap ON/OFF X or Y Amp?", f=w1793) -> (s? t:f=w1790:i16)
        n1261 = Select(t=w1793, s="Trap ON/OFF X or Y Amp?", f=w1796) -> (s? t:f=w1788:i16)
        n1262 = Select(t=w1793, s="Trap ON/OFF X or Y Amp?", f=w1795) -> (s? t:f=w1789:i16)
        n1263 = Select(t=w1793, s="Trap ON/OFF X or Y Amp?", f=w1794) -> (s? t:f=w1787:i16)
        n1264 = And(x="All FB On/Off", y="Feedback On/Off") -> (x .and. y?=w1785:cluster{"Set 1":bool, "Set 2":bool})
        n1265 = local read "BD 1 Amplitude 1 (%)"() -> (w1805:dbl)
        n1266 = local read "BD 1 Amplitude 2 (%)"() -> (w1804:dbl)
        n1267 = local read "BD 1 Amplitude 3 (%)"() -> (w1803:dbl)
        n1268 = Unbundle By Name(w1785) -> ("Set 1"=w1780:bool, "Set 2"=w1777:bool)
        n1269 = local read "Y RF Amplitude Limits (%)"() -> (w1773:T16)
        n1270 = local read "X RF Amplitude Limits (%)"() -> (w1774:T16)
        n1271 = local read "BD 2 Amplitude 1 (%)"() -> (w1806:dbl)
        n1272 = local read "BD 2 Amplitude 2 (%)"() -> (w1807:dbl)
        n1273 = local read "BD 2 Amplitude 3 (%)"() -> (w1808:dbl)
        n1274 = And(x="Trap 2 ON", y=w1777) -> (x .and. y?=w1775:bool)
        n1275 = And(x="Trap 1 ON", y=w1780) -> (x .and. y?=w1778:bool)
        n1276 = Multiply(x=w1792, y=w1805) -> (x*y=w1800:dbl)
        n1277 = Multiply(x=w1804, y=w1791) -> (x*y=w1798:dbl)
        n1278 = Multiply(x=w1803, y=w1790) -> (x*y=w1799:dbl)
        n1279 = Multiply(x=w1806, y=w1789) -> (x*y=w1809:dbl)
        n1280 = Multiply(x=w1807, y=w1788) -> (x*y=w1810:dbl)
        n1281 = Multiply(x=w1808, y=w1787) -> (x*y=w1811:dbl)
        n1282 = call "set RF board amplitude - interlace.vi"("Board 2 Amplitude Limits"=w1773, "Board 1 Amplitude Limits"=w1774, "error in"=w1801, "FPGA VI Reference In"=w1802, "Board 2 Amplitude 3 (%)"=w1811, "Board 1 Amplitude 3 (%)"=w1799, "Board 2 Amplitude 2 (%)"=w1810, "Board 2 Amplitude 1 (%)"=w1809, "Board 1 Amplitude 2 (%)"=w1798, "Board 1 Amplitude 1 (%)"=w1800) -> ("error out"=w1782:errorcluster, "FPGA VI Reference Out"=w1783:T20)
        n1283 = xnode "Read/Write Control"("FPGA VI Reference In"=w1783, "error in"=w1782, "FB On/Off Set 1"=w1778, "FB On/Off Set 2"=w1775) -> ("error out"=w1781:errorcluster)  [unwired: 1 out]
      }
      event "Load parameters": Value Change {
        n1284 = event-data() -> ()  [unwired: 7 out]
        n1285 = property on="Saved AOD Raster Scan Parameter Sets" class="Arr (strict)"() -> ("Index Values"=w1822:u32[])  [unwired: 2 in, 2 out]
        n1286 = Index Array(array=w1822, index=0) -> (element=w1819:u32)
        n1287 = local write "Load parameters"(FALSE ("Load parameters")) -> ()
        n1288 = Index Array(array="Saved AOD Raster Scan Parameter Sets", index=w1819) -> (element=w1818:T29)
        n1289 = Unbundle By Name(w1818) -> ("Scan Range AOD (nm) 2"=w1817:dbl, "Step Size AOD (nm) 2"=w1816:dbl, "Scan Speed AOD (nm/s) 2"=w1815:dbl, "Number of scans (AOD) 2"=w1814:u16)
        n1290 = flat-sequence {
          tunnel: w1817 -> [w1825]
          tunnel: w1816 -> [w1824]
          tunnel: w1815 -> [w1823]
          tunnel: w1814 -> [w1826]
          frame #0 {
            n1291 = local write "Scan Speed (nm/s)"(w1823) -> ()
            n1292 = local write "Scan Range (nm)"(w1825) -> ()
            n1293 = local write "Step Size (nm)"(w1824) -> ()
          }
          frame #1 {
            n1294 = property on="Number of F/B Scans (AOD)" class="DigNum (strict)"("Val(Sgnl)"=w1826) -> ()  [unwired: 2 in, 2 out]
          }
        }
      }
      event "Trap 1 (ON/OFF)", "Trap 2 (ON/OFF)": Value Change {
        n1295 = event-data() -> ()  [unwired: 7 out]
        n1296 = property on="Trap 2 ON" class="Bool (strict)"("Val(Sgnl)"="Trap 2 (ON/OFF)") -> ()  [unwired: 2 in, 2 out]
        n1297 = property on="Trap 1 ON" class="Bool (strict)"("Val(Sgnl)"="Trap 1 (ON/OFF)") -> ()  [unwired: 2 in, 2 out]
      }
      event "DIO count 1 (ticks)", "DIO count 2 (ticks)", "DIO count 3 (ticks)", "Interlace", "Number Interlace Sets", "Not-Interlacing Set": Value Change {
        n1298 = event-data() -> ()  [unwired: 7 out]
        n1299 = local read "DIO count 3 (ticks)"() -> (w1839:u16)
        n1300 = local read "DIO count 1 (ticks)"() -> (w1841:u16)
        n1301 = local read "DIO count 2 (ticks)"() -> (w1840:u16)
        n1302 = To Unsigned Byte Integer(number="Not-Interlacing Set") -> (unsigned 8bit integer=w1830:u8)
        n1303 = Add(x=w1830, y=u8 1) -> (x+y=w1834:u8)
        n1304 = xnode "Read/Write Control"("FPGA VI Reference In"=w1845, "error in"=w1843, "DIO count 1 (ticks)"=w1841, "DIO count 2 (ticks)"=w1840, "DIO count 3 (ticks)"=w1839, "Interlace ON/OFF"="Interlace", "Number Interlace Cycles"="Number Interlace Sets", "Interlace Off Parameters"=w1834) -> ("error out"=w1844:errorcluster)  [unwired: 1 out]
        n1305 = Build Array(w1841, w1840, w1839) -> (w1832:u16[])
        n1306 = Split 1D Array(array=w1832, index="Number Interlace Sets") -> (first subarray=w1842:u16[])  [unwired: 1 out]
        n1307 = Index Array(array=w1832, index=w1830) -> (element=w1831:u16)
        n1308 = Add Array Elements(numeric array=w1842) -> (sum=w1836:u16)
        n1309 = Select(t=w1836, s="Interlace", f=w1831) -> (s? t:f=→"Total Counts (ticks)":u16)
      }
      event "Reset Feedback": Value Change {
        n1310 = event-data() -> ()  [unwired: 7 out]
        n1311 = Unbundle By Name("Reset Feedback") -> ("Set 1"=w1849:bool, "Set 2"=w1848:bool)
        n1312 = xnode "Read/Write Control"("FPGA VI Reference In"=w1851, "error in"=w1846, "FB Reset Set 1"=w1849, "FB Reset Set 2"=w1848) -> ("error out"=w1847:errorcluster)  [unwired: 1 out]
      }
      event "Trap Intensity PID Gains": Value Change {
        n1313 = event-data() -> ()  [unwired: 7 out]
        n1314 = Unbundle By Name("Trap Intensity PID Gains") -> ("proportional gain (Kc)"=w1854:i16, "integral gain (Kc*Ts/Ti)"=w1853:i16, "derivative gain (Kc*Td/Ts)"=w1852:i16)
        n1315 = xnode "Read/Write Control"("FPGA VI Reference In"=w1858, "error in"=w1856, "P1"=w1854, "I1"=w1853, "D1"=w1852) -> ("error out"=w1857:errorcluster)  [unwired: 1 out]
      }
      event "AI2 to Setpoint", "Setpoints (V)": Value Change {
        n1316 = event-data() -> ()  [unwired: 7 out]
        n1317 = xnode "Read/Write Control"("FPGA VI Reference In"=w1863, "error in"=w1859) -> ("FPGA VI Reference Out"=w1862:T20, "error out"=w1861:errorcluster, "AI2 Y Sum Set 1"=w1870:i16, "AI2 Y Sum Set 2"=w1869:i16)
        n1318 = Cluster To Array(cluster="AI2 to Setpoint") -> (array=w1873:bool[])
        n1319 = local read "AI2 (V)"() -> (w1871:cluster{"Set 1":dbl, "Set 2":dbl})
        n1320 = Or Array Elements(Boolean array=w1873) -> (logical OR=w1874:bool)
        n1321 = Bundle By Name(cluster=w1871, "Set 1"=w1870, "Set 2"=w1869) -> (w1868:cluster{"Set 1":dbl, "Set 2":dbl})
        n1322 = Divide(x=w1868, y=3276.7) -> (x/y=w1867:cluster{"Set 1":dbl, "Set 2":dbl})
        "AI2 (V)" <- w1867
        n1323 = case shown="True" w1874 {
          tunnel: [w1877 w1894] -> w1866
          tunnel: "AI2 to Setpoint" -> [_ w1890]
          tunnel: "Setpoints (V)" -> [w1878 w1893]
          tunnel: w1867 -> [_ w1887]
          frame False {
            n1324 = Multiply(x=3276.7, y=w1878) -> (x*y=w1879:cluster{"Set 1":dbl, "Set 2":dbl})
            n1325 = To Word Integer(number=w1879) -> (16bit integer=w1877:cluster{"Set 1":i16, "Set 2":i16})
          }
          frame True {
            n1326 = Unbundle By Name(w1887) -> ("Set 1"=w1886:dbl, "Set 2"=w1885:dbl)
            n1327 = Unbundle By Name(w1893) -> ("Set 1"=w1892:dbl, "Set 2"=w1891:dbl)
            n1328 = Unbundle By Name(w1890) -> ("Set 1"=w1889:bool, "Set 2"=w1888:bool)
            n1329 = Select(t=w1886, s=w1889, f=w1892) -> (s? t:f=w1884:dbl)
            n1330 = Select(t=w1885, s=w1888, f=w1891) -> (s? t:f=w1883:dbl)
            n1331 = Bundle By Name(cluster=w1893, "Set 1"=w1884, "Set 2"=w1883) -> (w1881:cluster{"Set 1":dbl, "Set 2":dbl})
            n1332 = local write "Setpoints (V)"(w1881) -> ()
            n1333 = Multiply(x=3276.7, y=w1881) -> (x*y=w1882:cluster{"Set 1":dbl, "Set 2":dbl})
            n1334 = To Word Integer(number=w1882) -> (16bit integer=w1894:cluster{"Set 1":i16, "Set 2":i16})
          }
        }
        n1335 = Unbundle By Name(w1866) -> ("Set 1"=w1865:i16, "Set 2"=w1864:i16)
        n1336 = xnode "Read/Write Control"("FPGA VI Reference In"=w1862, "error in"=w1861, "FB Setpoint Set 1"=w1865, "FB Setpoint Set 2"=w1864) -> ("error out"=w1860:errorcluster)  [unwired: 1 out]
      }
      event "+ phase (GI)", "- phase (GI)", "+ phase (GI) 2", "- phase (GI) 2", "+ phase (RI)", "- phase (RI)", "+ phase (RI) 2", "- phase (RI) 2", "+ phase (Green FB)", "- phase (Green FB)", "+ phase (RI FB)", "- phase (RI FB)": Value Change {
        n1337 = event-data() -> ()  [unwired: 7 out]
        n1338 = Or(x="+ phase (GI)", y="- phase (GI)") -> (x .or. y?=w1947:bool)
        n1339 = Negate(x="Phase adj. (GI)") -> (-x=w1952:i16)
        n1340 = Select(t=w1952, s="+ phase (GI)", f="Phase adj. (GI)") -> (s? t:f=w1951:i16)
        n1341 = Or(x="+ phase (GI) 2", y="- phase (GI) 2") -> (x .or. y?=w1938:bool)
        n1342 = Negate(x="Phase adj. (GI) 2") -> (-x=w1943:i16)
        n1343 = Select(t=w1943, s="+ phase (GI) 2", f="Phase adj. (GI) 2") -> (s? t:f=w1939:i16)
        n1344 = Negate(x="Phase adj. (RI)") -> (-x=w1937:i16)
        n1345 = Or(x="+ phase (RI)", y="- phase (RI)") -> (x .or. y?=w1933:bool)
        n1346 = Select(t=w1937, s="+ phase (RI)", f="Phase adj. (RI)") -> (s? t:f=w1932:i16)
        n1347 = Negate(x="Phase adj. (RI) 2") -> (-x=w1931:i16)
        n1348 = Or(x="+ phase (RI) 2", y="- phase (RI) 2") -> (x .or. y?=w1920:bool)
        n1349 = Select(t=w1931, s="+ phase (RI) 2", f="Phase adj. (RI) 2") -> (s? t:f=w1927:i16)
        n1350 = Or(x="+ phase (Green FB)", y="- phase (Green FB)") -> (x .or. y?=w1921:bool)
        n1351 = Negate(x="Phase adj. (Green FB)") -> (-x=w1926:i16)
        n1352 = Select(t=w1926, s="+ phase (Green FB)", f="Phase adj. (Green FB)") -> (s? t:f=w1922:i16)
        n1353 = Or(x="+ phase (RI FB)", y="- phase (RI FB)") -> (x .or. y?=w1914:bool)
        n1354 = Negate(x="Phase adj. (RI FB)") -> (-x=w1919:i16)
        n1355 = Select(t=w1919, s="+ phase (RI FB)", f="Phase adj. (RI FB)") -> (s? t:f=w1915:i16)
        n1356 = Negate(x="Phase adj. (BI AO)") -> (-x=w1913:i16)
        n1357 = Or(x="+ phase (BI AO)", y="- phase (BI AO)") -> (x .or. y?=w1898:bool)
        n1358 = Select(t=w1913, s="+ phase (BI AO)", f="Phase adj. (BI AO)") -> (s? t:f=w1901:i16)
        n1359 = Negate(x="Phase adj. (BI DO)") -> (-x=w1909:i16)
        n1360 = Or(x="+ phase (BI DO)", y="- phase (BI DO)") -> (x .or. y?=w1897:bool)
        n1361 = Select(t=w1909, s="+ phase (BI DO)", f="Phase adj. (BI DO)") -> (s? t:f=w1900:i16)
        n1362 = Negate(x="Phase adj. (BI AI)") -> (-x=w1905:i16)
        n1363 = Or(x="+ phase (BI AI)", y="- phase (BI AI)") -> (x .or. y?=w1896:bool)
        n1364 = Select(t=w1905, s="+ phase (BI AI)", f="Phase adj. (BI AI)") -> (s? t:f=w1899:i16)
        n1365 = xnode "Read/Write Control"("FPGA VI Reference In"=w1954, "error in"=w1953, "Phase count adjustment (GI)"=w1951, "Phase count adjustment (GI) 2"=w1939, "Phase count adjustment (RI)"=w1932, "Phase count adjustment (RI) 2"=w1927, "Phase count adjustment (Green FB)"=w1922, "Phase count adjustment (Red FB)"=w1915, "Phase count adjustment (BI AO)"=w1901, "Phase count adjustment (BI D)"=w1900, "Phase count adjustment (Blue Int)"=w1899) -> ("FPGA VI Reference Out"=w1949:T20, "error out"=w1950:errorcluster)
        n1366 = xnode "Read/Write Control"("FPGA VI Reference In"=w1949, "error in"=w1950, "+ phase (GI)"=w1947, "+ phase (GI) 2"=w1938, "+ phase (RI)"=w1933, "+ phase (RI) 2"=w1920, "+ phase (Green FB)"=w1921, "+ phase (Red FB)"=w1914, "+ phase (BI AO)"=w1898, "+ phase (BI D)"=w1897, "+ phase (Blue Int)"=w1896) -> ("error out"=w1948:errorcluster)  [unwired: 1 out]
      }
      event "Green Laser ON/OFF", "Red Laser ON/OFF", "Blue Laser ON/OFF": Value Change {
        # "This loop shouldn't be initialized.  The main 'laser ON' settings should dominate and set the others."
        n1367 = event-data() -> ()  [unwired: 7 out]
        n1368 = property on="Red Laser ON" class="Bool (strict)"("Val(Sgnl)"="Red Laser ON/OFF") -> ()  [unwired: 2 in, 2 out]
        n1369 = property on="Blue Laser ON" class="Bool (strict)"("Val(Sgnl)"="Blue Laser ON/OFF") -> ()  [unwired: 2 in, 2 out]
        n1370 = property on="Green Laser ON" class="Bool (strict)"("Val(Sgnl)"="Green Laser ON/OFF") -> ()  [unwired: 2 in, 2 out]
      }
      event "Laser interlacing mode", "Green Laser ON", "Red Laser ON", "Blue Laser ON": Value Change {
        n1371 = event-data() -> ()  [unwired: 7 out]
        n1372 = local write "Green Laser ON/OFF"("Green Laser ON") -> ()
        n1373 = local write "Blue Laser ON/OFF"("Blue Laser ON") -> ()
        n1374 = local write "Red Laser ON/OFF"("Red Laser ON") -> ()
        n1375 = case shown="True" "Green Laser ON" {
          tunnel: "Laser interlacing mode" -> [_ w1991]
          tunnel: [enum32{"Laser ON", "Laser OFF", "Interlace"}."Laser OFF" ("Green laser mode") w1991] -> w1967
          tunnel: [FALSE w1987] -> w1966
          frame False {
          }
          frame True {
            n1376 = local read "Green FB On/Off"() -> (w1988:bool)
            n1377 = Equal?(x=w1991, y=enum32{"Laser ON", "Laser OFF", "Interlace"}."Interlace") -> (x = y?=w1989:bool)
            n1378 = And(x=w1989, y=w1988) -> (x .and. y?=w1987:bool)
          }
        }
        n1379 = case shown="True" "Red Laser ON" {
          tunnel: "Laser interlacing mode" -> [_ w1984]
          tunnel: [enum32{"Laser ON", "Laser OFF", "Interlace"}."Laser OFF" ("Green laser mode") w1984] -> w1963
          tunnel: [FALSE w1980] -> w1962
          frame False {
          }
          frame True {
            n1380 = local read "Red FB On/Off"() -> (w1981:bool)
            n1381 = Equal?(x=w1984, y=enum32{"Laser ON", "Laser OFF", "Interlace"}."Interlace") -> (x = y?=w1982:bool)
            n1382 = And(x=w1982, y=w1981) -> (x .and. y?=w1980:bool)
          }
        }
        n1383 = case shown="True" "Blue Laser ON" {
          tunnel: "Laser interlacing mode" -> [_ w1975]
          tunnel: [enum32{"Laser ON", "Laser OFF", "Interlace"}."Laser OFF" ("Green laser mode") w1975] -> w1959
          tunnel: [FALSE w1973] -> w1958
          frame False {
          }
          frame True {
            n1384 = local read "Blue FB On/Off"() -> (w1974:bool)
            n1385 = Equal?(x=w1975, y=enum32{"Laser ON", "Laser OFF", "Interlace"}."Interlace") -> (x = y?=w1976:bool)
            n1386 = And(x=w1976, y=w1974) -> (x .and. y?=w1973:bool)
          }
        }
        n1387 = xnode "Read/Write Control"("FPGA VI Reference In"=w1970, "error in"=w1968, "Operating Mode"=w1967, "Operating Mode 2"=w1967, "Green FB On/Off"=w1966, "Red Laser Operating Mode"=w1963, "RI Operating Mode 2"=w1963, "Red FB On/Off"=w1962, "BI Operating Mode (AO)"=w1959, "Blue Laser Operating Mode (D)"=w1959, "Blue FB On/Off"=w1958) -> ("error out"=w1969:errorcluster)  [unwired: 1 out]
      }
      event "Invert laser interlacing": Value Change {
        n1388 = event-data() -> ()  [unwired: 7 out]
        n1389 = xnode "Read/Write Control"("FPGA VI Reference In"=w1995, "error in"=w1993, "Invert GI"="Invert laser interlacing", "Invert GI 2"="Invert laser interlacing", "Invert RI"="Invert laser interlacing", "Invert RI 2"="Invert laser interlacing", "Invert BI (AO)"="Invert laser interlacing", "Invert BI (D)"="Invert laser interlacing") -> ("error out"=w1994:errorcluster)  [unwired: 1 out]
      }
      event "Green FB Setpoint (mV)", "Green FB Gains", "Green FB On/Off", "Green Intensity % (FB OFF)", "Green int current ON count adj": Value Change {
        n1390 = event-data() -> ()  [unwired: 7 out]
        n1391 = local read "Green FB Setpoint (mV)"() -> (w2006:dbl)
